vi "Vision Processing.vi"(4 "error in (no error)":errorcluster) -> ()   [LabVIEW 2012]
doc: "This VI runs in parallel to other tasks. It gets images from the camera, processes them for color or shape and use that information to affect robot behavior."
uses:
  Robot Global Data.vi
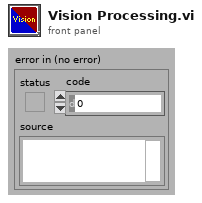
[diagram p1: front panel]
types:
  T1 = typedef "WPI_CameraDevRef.ctl" = cluster{"Camera Address":string, "CameraStatus":errorcluster, "Acquire Image Notifier":refnum<notifier>}
  T2 = typedef "WPI_CameraImageSize.ctl" = enum16{"640x480", "320x240", "160x120"}
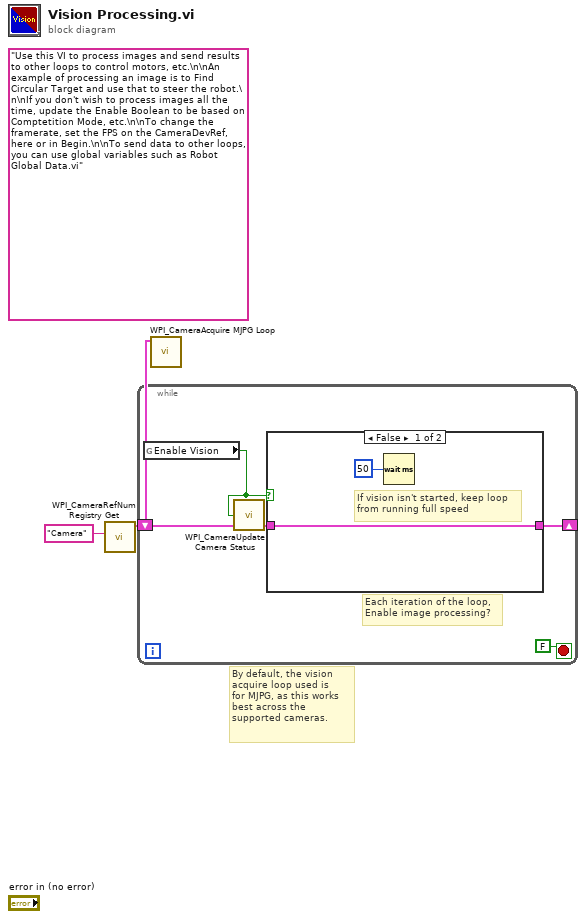
[diagram p0: block diagram]
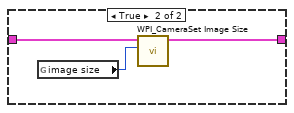
[diagram p2: hidden frame]
diagram:
  (unwired) "Use this VI to process images and send results to other loops to control motors, etc.\n\nAn example of processing an image is to Find Circular Target and use that to steer the robot.\n\nIf you don't wish to process images all the time, update the Enable Boolean to be based on Comptetition Mode, etc.\n\nTo change the framerate, set the FPS on the CameraDevRef, here or in Begin.\n\nTo send data to other loops, you can use global variables such as Robot Global Data.vi"
  # "By default, the vision\nacquire loop used is\nfor MJPG, as this works\nbest across the\nsupported cameras."
  n1 = call <vilib>:"WPI_CameraRefNum Registry Get.vi"("refnum name"="Camera") -> ("CameraDevRef"=w1:T1)  [unwired: 1 in, 9 out]
  n2 = while {
    shift-right: [w6] -> _
    shift-left: w1 -> [w5]
    stop <- FALSE stop-if-true
    # "Each iteration of the loop,\nEnable image processing?"
    n3 = global read "Robot Global Data.vi" "Enable Vision"() -> (w3:bool)
    n4 = call <vilib>:"WPI_CameraUpdate Camera Status.vi"("CameraDevRef In"=w5, "Enable Vision"=w3) -> ("CameraDevRef Out"=w4:T1)  [unwired: 3 in]
    n5 = case shown="False" w3 {
      tunnel: [w9 w12] -> w6
      tunnel: w4 -> [w9 w11]
      frame False {
        # "If vision isn't started, keep loop\nfrom running full speed"
        n6 = Wait (ms)(milliseconds to wait=u32 50) -> ()  [unwired: 1 out]
      }
      frame True {
        n7 = global read "Robot Global Data.vi" "image size"() -> (w10:T2)
        n8 = call <vilib>:"WPI_CameraSet Image Size.vi"("Image Size"=w10, "CameraDevRef"=w11) -> ("CameraDevRef Out"=w12:T1)  [unwired: 1 in, 8 out]
      }
    }
  }
  n9 = call <vilib>:"WPI_CameraAcquire MJPG Loop.vi"("CameraDevRef"=w1) -> ()  [unwired: 11 in]
